vi "FPGA_AIReadLoopTiming.vi"(8 "error in (no error)":errorcluster, 11 "AI Reference":T1) -> (0 "error out":errorcluster, 2 "LoopTiming":u32, 3 "AI Reference":T1)   [LabVIEW 2017]
uses:
  <vilib>/Rock Robotics/SystemInterfaces/AI/FPGA_AIDevRef.ctl
  <vilib>/Rock Robotics/SystemInterfaces/System/FPGA_SystemFPGA Ref Global.vi
  <vilib>/Utility/error.llb/Error Cluster From Error Code.vi
  <vilib>/rvi/errors/niLvFpgaAdjustHostInterfaceError.vi
  <vilib>/rvi/interface/nirviReadWriteControl/nirviReadWriteControl.xnode
  <vilib>/Rock Robotics/SystemInterfaces/System/FPGA_SystemFRC FPGA Ref.ctl
  NiFpgaLv.dll
  <vilib>/rvi/interface/Simulation/niFpgaSimulationCallBeginRW.vi
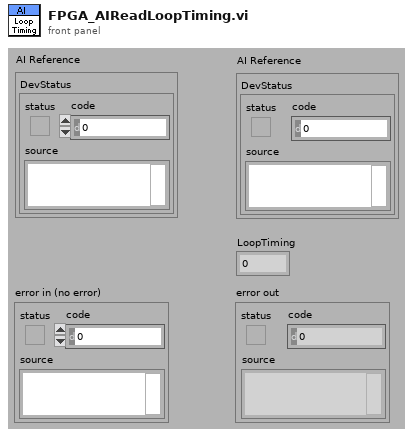
[diagram p1: front panel]
types:
  T1 = typedef "FPGA_AIDevRef.ctl" = cluster{"DevStatus":errorcluster}
  T2 = typedef "FPGA_SystemFRC FPGA Ref.ctl" = refnum<k20>
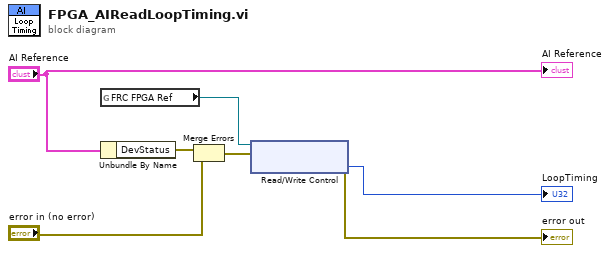
[diagram p0: block diagram]
diagram:
  n1 = global read "FPGA_SystemFPGA Ref Global.vi" "FRC FPGA Ref"() -> (w4:T2)
  n2 = Unbundle By Name("AI Reference") -> ("DevStatus"=w3:errorcluster)
  n3 = Merge Errors(w3, "error in (no error)") -> (w2:errorcluster)
  n4 = xnode "Read/Write Control"("FPGA VI Reference In"=w4, "error in"=w2) -> ("error out"=→"error out":errorcluster, "AI.LoopTiming"=→"LoopTiming":u32)  [unwired: 1 out]
  "AI Reference" <- "AI Reference"
